vi "温度标定.vi"(11 "输入电压":dbl) -> (3 "输出温度":dbl)   [LabVIEW 2016]
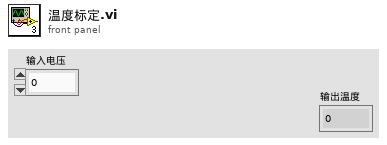
[diagram p1: front panel]
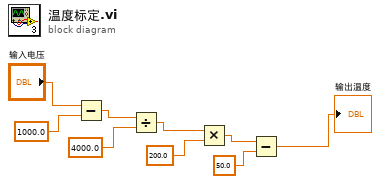
[diagram p0: block diagram]
diagram:
  n1 = Subtract(x="输入电压", y=1000.0) -> (x-y=w7:dbl)
  n2 = Divide(x=w7, y=4000.0) -> (x/y=w5:dbl)
  n3 = Multiply(x=w5, y=200.0) -> (x*y=w3:dbl)
  n4 = Subtract(x=w3, y=50.0) -> (x-y=→"输出温度":dbl)
